vi "color_front_pannel.vi"() -> (2 "Resolved Color":u32)   [LabVIEW 2014]
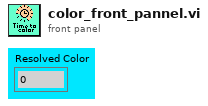
[diagram p1: front panel]
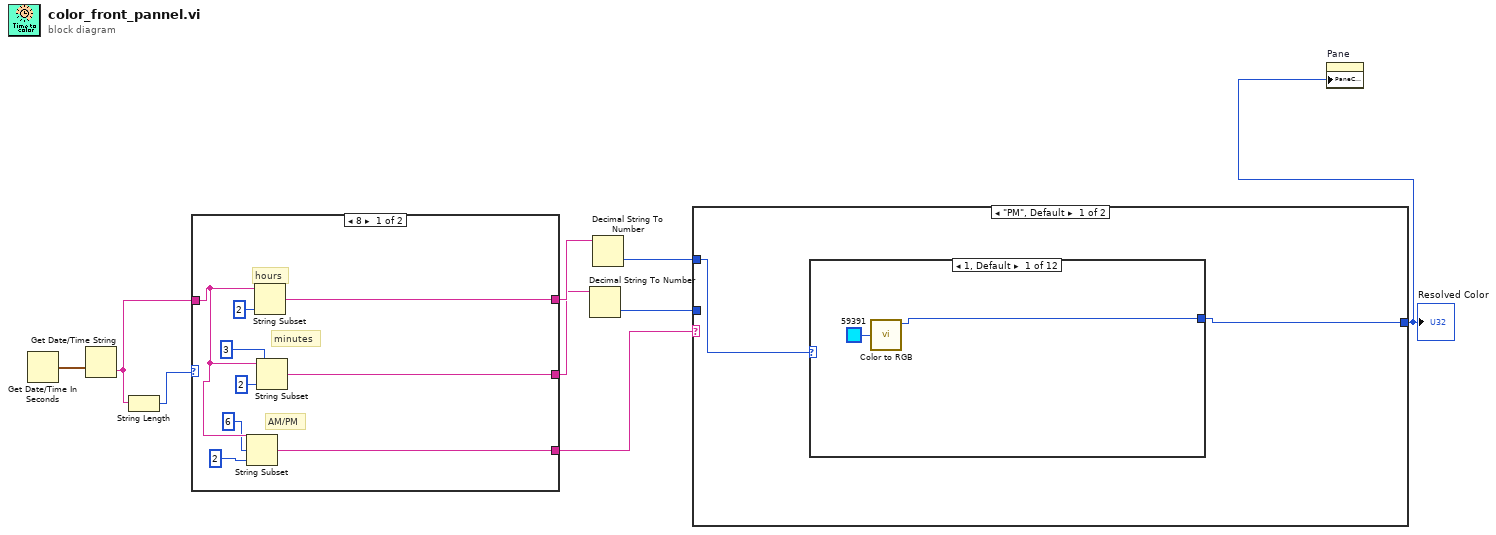
[diagram p0: block diagram]
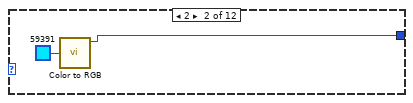
[diagram p2: hidden frame]
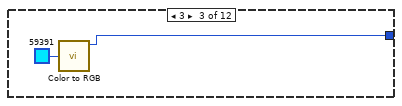
[diagram p3: hidden frame]
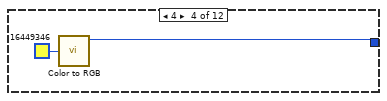
[diagram p4: hidden frame]
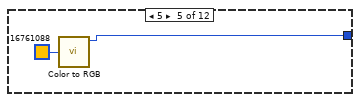
[diagram p5: hidden frame]
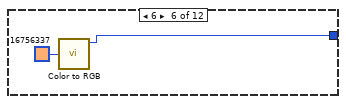
[diagram p6: hidden frame]
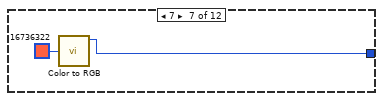
[diagram p7: hidden frame]
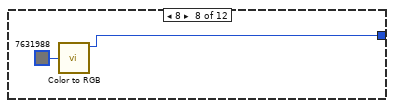
[diagram p8: hidden frame]
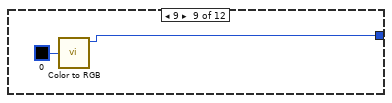
[diagram p9: hidden frame]
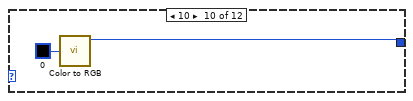
[diagram p10: hidden frame]
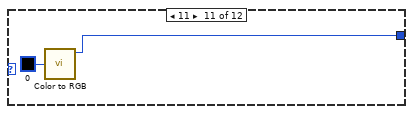
[diagram p11: hidden frame]
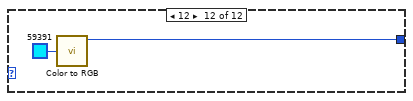
[diagram p12: hidden frame]
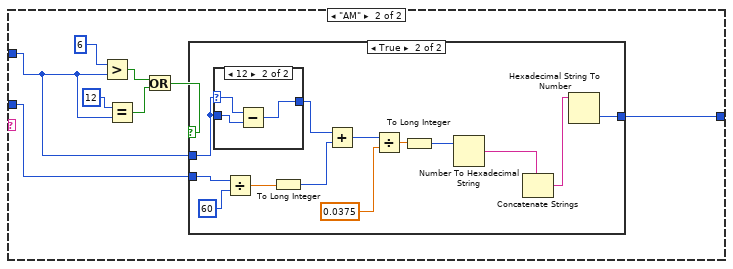
[diagram p13: hidden frame]
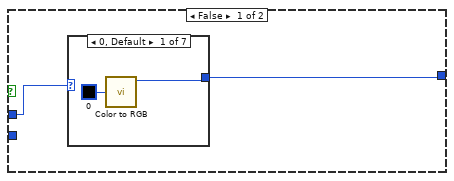
[diagram p14: hidden frame]
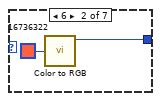
[diagram p15: hidden frame]
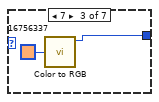
[diagram p16: hidden frame]
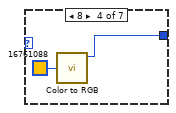
[diagram p17: hidden frame]
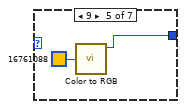
[diagram p18: hidden frame]
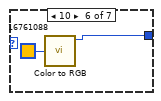
[diagram p19: hidden frame]
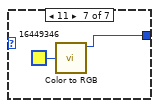
[diagram p20: hidden frame]
diagram:
  n1 = Get Date/Time In Seconds() -> (seconds since 1Jan1904=w9:timestamp)
  n2 = Get Date/Time String(seconds (now)=w9) -> (time string=w7:string)  [unwired: 2 in, 1 out]
  n3 = String Length(string=w7) -> (length=w8:i32)
  n4 = case shown="8" w8 {
    tunnel: w7 -> [w14 w22]
    tunnel: [w12 w21] -> w6
    tunnel: [w11 w20] -> w5
    tunnel: [w10 w19] -> w4
    frame 8 {
      # "AM/PM"
      # "minutes"
      # "hours"
      n5 = String Subset(string=w14, offset (0)=6, length (rest)=2 ("length (rest)")) -> (substring=w10:string)
      n6 = String Subset(string=w14, length (rest)=2 ("length (rest)")) -> (substring=w12:string)  [unwired: 1 in]
      n7 = String Subset(string=w14, offset (0)=3, length (rest)=2 ("length (rest)")) -> (substring=w11:string)
    }
    frame 7, Default {
      # "AM/PM"
      # "minutes"
      # "hours"
      n8 = String Subset(string=w22, offset (0)=5, length (rest)=2 ("length (rest)")) -> (substring=w19:string)
      n9 = String Subset(string=w22, length (rest)=1 ("length (rest)")) -> (substring=w21:string)  [unwired: 1 in]
      n10 = String Subset(string=w22, offset (0)=2, length (rest)=2 ("length (rest)")) -> (substring=w20:string)
    }
  }
  n11 = Decimal String To Number(string=w5) -> (number=w2:i32)  [unwired: 2 in, 1 out]
  n12 = Decimal String To Number(string=w6) -> (number=w3:i32)  [unwired: 2 in, 1 out]
  n13 = case shown="\"PM\", Default" w4 {
    tunnel: w3 -> [w29 w56]
    tunnel: w2 -> [_ w55]
    tunnel: [w28 w54] -> w1
    frame "PM", Default {
      n14 = case shown="1, Default" w29 {
        tunnel: [w30 w32 w34 w36 w38 w40 w42 w44 w46 w48 w50 w52] -> w28
        frame 1, Default {
          n15 = call <vilib>:"Color to RGB.vi"("Color"=u32 59391) -> ("Resolved Color"=w30:u32)  [unwired: 3 out]
        }
        frame 2 {
          n16 = call <vilib>:"Color to RGB.vi"("Color"=u32 59391) -> ("Resolved Color"=w32:u32)  [unwired: 3 out]
        }
        frame 3 {
          n17 = call <vilib>:"Color to RGB.vi"("Color"=u32 59391) -> ("Resolved Color"=w34:u32)  [unwired: 3 out]
        }
        frame 4 {
          n18 = call <vilib>:"Color to RGB.vi"("Color"=u32 16449346) -> ("Resolved Color"=w36:u32)  [unwired: 3 out]
        }
        frame 5 {
          n19 = call <vilib>:"Color to RGB.vi"("Color"=u32 16761088) -> ("Resolved Color"=w38:u32)  [unwired: 3 out]
        }
        frame 6 {
          n20 = call <vilib>:"Color to RGB.vi"("Color"=u32 16756337) -> ("Resolved Color"=w40:u32)  [unwired: 3 out]
        }
        frame 7 {
          n21 = call <vilib>:"Color to RGB.vi"("Color"=u32 16736322) -> ("Resolved Color"=w42:u32)  [unwired: 3 out]
        }
        frame 8 {
          n22 = call <vilib>:"Color to RGB.vi"("Color"=u32 7631988) -> ("Resolved Color"=w44:u32)  [unwired: 3 out]
        }
        frame 9 {
          n23 = call <vilib>:"Color to RGB.vi"("Color"=u32 0) -> ("Resolved Color"=w46:u32)  [unwired: 3 out]
        }
        frame 10 {
          n24 = call <vilib>:"Color to RGB.vi"("Color"=u32 0) -> ("Resolved Color"=w48:u32)  [unwired: 3 out]
        }
        frame 11 {
          n25 = call <vilib>:"Color to RGB.vi"("Color"=u32 0) -> ("Resolved Color"=w50:u32)  [unwired: 3 out]
        }
        frame 12 {
          n26 = call <vilib>:"Color to RGB.vi"("Color"=u32 59391) -> ("Resolved Color"=w52:u32)  [unwired: 3 out]
        }
      }
    }
    frame "AM" {
      n27 = Greater?(x=6, y=w56) -> (0:w59:bool)
      n28 = Equal?(x=12, y=w56) -> (x = y?=w58:bool)
      n29 = Or(x=w59, y=w58) -> (x .or. y?=w57:bool)
      n30 = case shown="True" w57 {
        tunnel: w56 -> [w63 w90]
        tunnel: w55 -> [_ w89]
        tunnel: [w62 w78] -> w54
        frame False {
          n31 = case shown="0, Default" w63 {
            tunnel: [w64 w66 w68 w70 w72 w74 w76] -> w62
            frame 0, Default {
              n32 = call <vilib>:"Color to RGB.vi"("Color"=u32 0) -> ("Resolved Color"=w64:u32)  [unwired: 3 out]
            }
            frame 6 {
              n33 = call <vilib>:"Color to RGB.vi"("Color"=u32 16736322) -> ("Resolved Color"=w66:u32)  [unwired: 3 out]
            }
            frame 7 {
              n34 = call <vilib>:"Color to RGB.vi"("Color"=u32 16756337) -> ("Resolved Color"=w68:u32)  [unwired: 3 out]
            }
            frame 8 {
              n35 = call <vilib>:"Color to RGB.vi"("Color"=u32 16761088) -> ("Resolved Color"=w70:u32)  [unwired: 3 out]
            }
            frame 9 {
              n36 = call <vilib>:"Color to RGB.vi"("Color"=u32 16761088) -> ("Resolved Color"=w72:u32)  [unwired: 3 out]
            }
            frame 10 {
              n37 = call <vilib>:"Color to RGB.vi"("Color"=u32 16761088) -> ("Resolved Color"=w74:u32)  [unwired: 3 out]
            }
            frame 11 {
              n38 = call <vilib>:"Color to RGB.vi"("Color"=u32 16449346) -> ("Resolved Color"=w76:u32)  [unwired: 3 out]
            }
          }
        }
        frame True {
          n39 = case shown="12" w90 {
            selector: w90 -> [_ w94]
            tunnel: w90 -> [w91 w93]
            tunnel: [w91 w92] -> w87
            frame 0, Default {
            }
            frame 12 {
              n40 = Subtract(x=w94, y=w93) -> (x-y=w92:i32)
            }
          }
          n41 = Divide(x=w89, y=60) -> (x/y=w86:dbl)
          n42 = To Long Integer(number=w86) -> (32bit integer=w85:i32)
          n43 = Add(x=w87, y=w85) -> (x+y=w84:i32)
          n44 = Divide(x=w84, y=0.0375) -> (x/y=w82:dbl)
          n45 = To Long Integer(number=w82) -> (32bit integer=w81:i32)
          n46 = Number To Hexadecimal String(2:w81) -> (0:w80:string)  [unwired: 1 in]
          n47 = Concatenate Strings(w80, w80, w80) -> (w79:string)
          n48 = Hexadecimal String To Number(string=w79) -> (number=w78:u32)  [unwired: 2 in, 1 out]
        }
      }
    }
  }
  "Resolved Color" <- w1
  n49 = property on="Pane" class="Pane"("PaneColor"=w1) -> ()  [unwired: 2 in, 2 out]
